vi "Convert to NEC.vi"(10 "Error Interface in":refnum<class "Error Interface.lvclass">) -> (2 "error out":errorcluster)   [LabVIEW 2016, in "Stream Error.lvlib" / "Error Interface.lvclass"]
doc: "--\nCopyright © 2017 Composed SystemsI All rights reserved.\n\nAuthor: Jon McBee <jon.mcbee@composed.io>\n\nThis library is provided \"AS IS\" ,WITHOUT WARRANTIES OR\nCONDITIONS OF ANY KIND, either express or implied.\n\nComposed Systems -- composed.io\n\nStream 0.0.1.1\nJon McBee - Composed Systems\nCopyright (c) 2017, Composed Systems"
uses:
  <userlib>/Composed Systems/Stream/Error/Classes/Error Interface/Error Interface.lvclass
  <userlib>/Composed Systems/Stream/Error/Classes/Error Interface/Error Codes.ctl
  <userlib>/Composed Systems/Stream/Error/Classes/Error Interface/Error UID.ctl
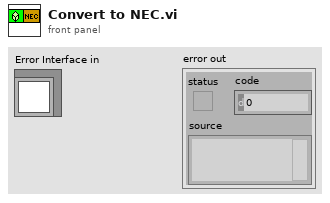
[diagram p1: front panel]
types:
  T1 = typedef "Stream Error.lvlib/Error Interface.lvclass/Error Codes.ctl" = enum16{"Invalid NEC Payload"}
  T2 = typedef "Stream Error.lvlib/Error Interface.lvclass/Error UID.ctl" = u16
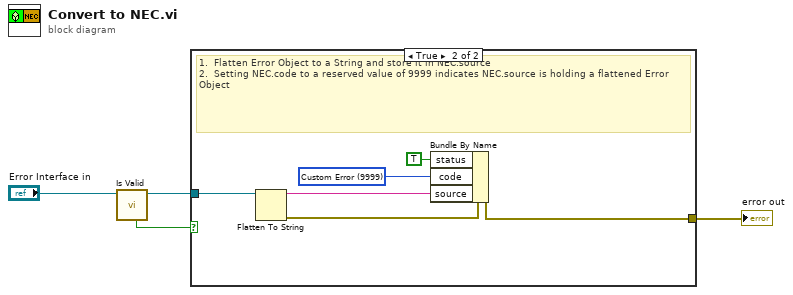
[diagram p0: block diagram]
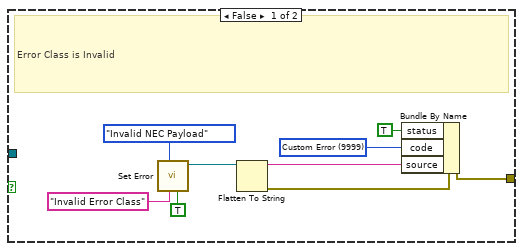
[diagram p2: hidden frame]
diagram:
  n1 = call <userlib>:"Is Valid.vi"("Error Interface in"="Error Interface in") -> ("Error Interface out"=w2:refnum<class "Error Interface.lvclass">, "Valid?"=w3:bool)  [unwired: 9 in]
  n2 = case shown="True" w3 {
    tunnel: w2 -> [_ w19]
    tunnel: [w5 w17] -> w1
    frame False {
      w8 = T2 9999 items=["Custom Error"=9999] ("Custom Error Codes")
      # "Error Class is Invalid"
      n3 = call <userlib>:"Set Error.vi"("Log Error?"=TRUE, "Error Message"="Invalid Error Class", "Error Codes"=Error_Codes."Invalid NEC Payload") -> ("Error Interface out"=w6:refnum<class "Error Interface.lvclass">)  [unwired: 8 in]
      n4 = Flatten To String(anything=w6) -> (data string=w7:string, error out=w10:errorcluster)  [unwired: 3 in, 1 out]
      n5 = Bundle By Name(cluster=w10, "status"=TRUE, "code"=w8, "source"=w7) -> (w5:errorcluster)
    }
    frame True {
      w15 = T2 9999 items=["Custom Error"=9999] ("Custom Error Codes")
      # "1.  Flatten Error Object to a String and store it in NEC.source\n2.  Setting NEC.code to a reserved value of 9999 indicates NEC.source is holding a flattened Error Object"
      n6 = Flatten To String(anything=w19) -> (data string=w14:string, error out=w18:errorcluster)  [unwired: 3 in, 1 out]
      n7 = Bundle By Name(cluster=w18, "status"=TRUE, "code"=w15, "source"=w14) -> (w17:errorcluster)
    }
  }
  "error out" <- w1
